vi "Configure Bus Source (Parallel).vi"(5 "Clock Source (23:Digital Channel 15)":u16(ring)=23 items=["Channel 1", "Channel 2", "Channel 3", "Channel 4", "Math 1", "Math 2", "Math 3", "Math 4", "Digital Channel 0", "Digital Channel 1", "Digital Channel 2", "Digital Channel 3", "Digital Channel 4", "Digital Channel 5", "Digital Channel 6", "Digital Channel 7", "Digital Channel 8", "Digital Channel 9", "Digital Channel 10", "Digital Channel 11", "Digital Channel 12", "Digital Channel 13", "Digital Channel 14", "Digital Channel 15"], 6 "Sources List":string, 7 "Enable Clocked (F:Disable)":bool, 8 "error in (no error)":errorcluster, 9 "Edge Type (0: Rise)":i32(ring) items=["Rise", "Fall", "Either"], 10 "BUS Number (0:Bus 1)":u8(ring) items=["Bus 1", "Bus 2", "Bus 3", "Bus 4", "Bus 5", "Bus 6", "Bus 7", "Bus 8", "Bus 9", "Bus 10", "Bus 11", "Bus 12", "Bus 13", "Bus 14", "Bus 15", "Bus 16"], 11 "VISA resource name":refnum<visa-resource-name>) -> (0 "error out":errorcluster, 3 "VISA resource name out":refnum<visa-resource-name>)   [LabVIEW 2011, in "Tektronix 7000 Series.lvlib"]
doc: "Configures Parallel Bus Setting for an oscilloscope."
uses:
  Tektronix 7000 Series.lvlib
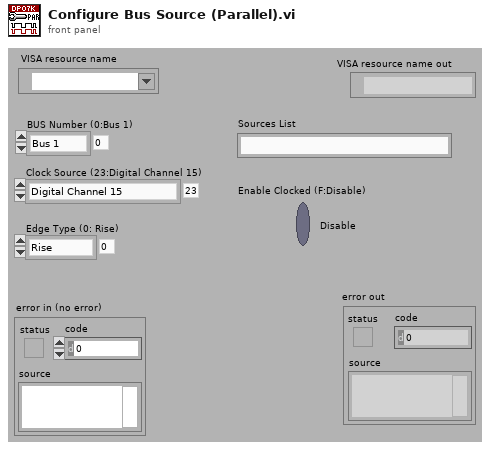
[diagram p1: front panel]
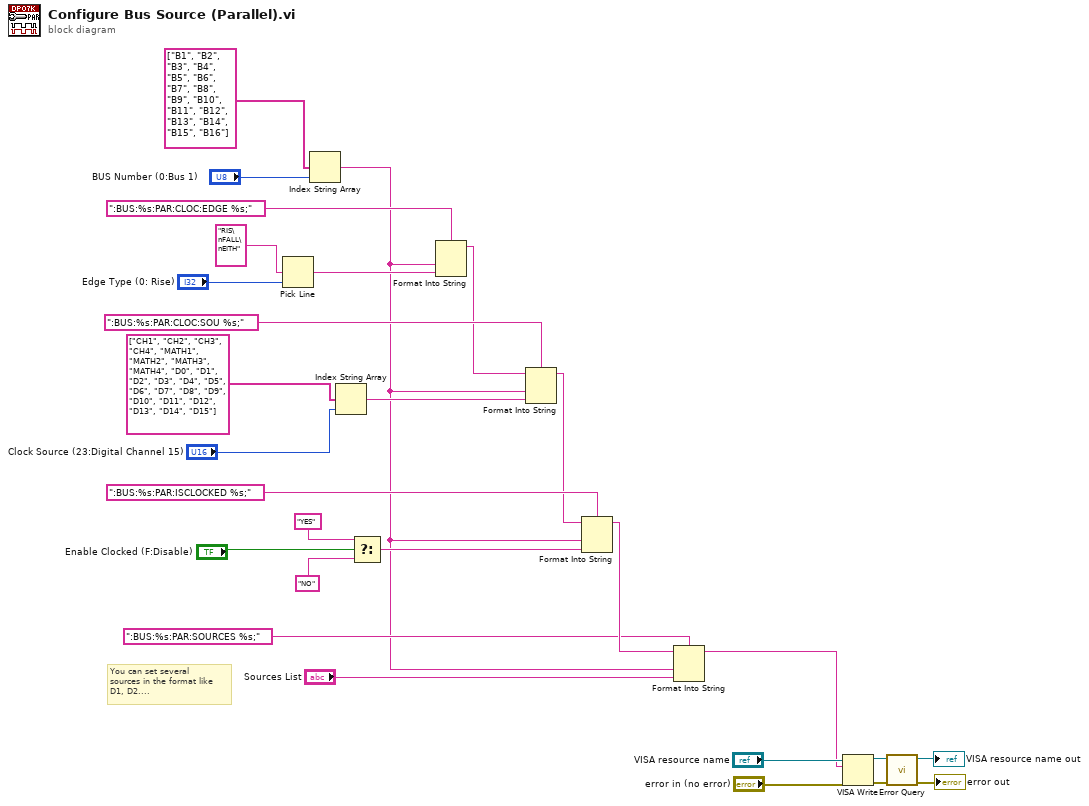
[diagram p0: block diagram]
diagram:
  # "You can set several\nsources in the format like\nD1, D2...."
  n1 = Pick Line(multi-line string="RIS\nFALL\nEITH", line index="Edge Type (0: Rise)") -> (output string=w26:string)  [unwired: 1 out]
  n2 = Index String Array(1:"BUS Number (0:Bus 1)", 2:string[] ["B1", "B2", "B3", "B4", "B5", "B6", "B7", "B8", "B9", "B10", "B11", "B12", "B13", "B14", "B15", "B16"]) -> (0:w3:string)  [unwired: 1 out]
  n3 = Index String Array(1:"Clock Source (23:Digital Channel 15)", 2:string[] ["CH1", "CH2", "CH3", "CH4", "MATH1", "MATH2", "MATH3", "MATH4", "D0", "D1", "D2", "D3", "D4", "D5", "D6", "D7", "D8", "D9", "D10", "D11", "D12", "D13", "D14", "D15"]) -> (0:w21:string)  [unwired: 1 out]
  n4 = Select(t="YES", s="Enable Clocked (F:Disable)", f="NO") -> (s? t:f=w14:string)
  n5 = Format Into String(format string=":BUS:%s:PAR:CLOC:EDGE %s;", w3, w26) -> (resulting string=w19:string)  [unwired: 2 in, 1 out]
  n6 = Format Into String(format string=":BUS:%s:PAR:CLOC:SOU %s;", initial string=w19, w3, w21) -> (resulting string=w18:string)  [unwired: 1 in, 1 out]
  n7 = Format Into String(format string=":BUS:%s:PAR:ISCLOCKED %s;", initial string=w18, w3, w14) -> (resulting string=w8:string)  [unwired: 1 in, 1 out]
  n8 = Format Into String(format string=":BUS:%s:PAR:SOURCES %s;", initial string=w8, w3, "Sources List") -> (resulting string=w4:string)  [unwired: 1 in, 1 out]
  n9 = VISA Write(VISA resource name="VISA resource name", write buffer=w4, error in (no error)="error in (no error)") -> (VISA resource name out=w11:refnum<visa-resource-name>, error out=w12:errorcluster)  [unwired: 1 out]
  n10 = call "Error Query.vi"("error in (no error)"=w12, "VISA resource name"=w11) -> ("error out"=→"error out":errorcluster, "VISA resource name out"=→"VISA resource name out":refnum<visa-resource-name>)  [unwired: 8 out]
